vi "Stages and Lasers Control Loop.vi"(8 "error in (no error)":errorcluster, 9 "DataNotifier":refnum<notifier>[](array[refnum]), 10 "DataQueues":refnum<queue>[](array[refnum]), 11 "Message Queues":T1) -> (0 "error out":errorcluster, 1 "DataNotifier Out":refnum<notifier>[](array[refnum]), 2 "DataQueues Out":refnum<queue>[](array[refnum]))   [LabVIEW 2019, in "Acquisition.lvlib"]
doc: "Message loop for handling messages pertaining to the acquisition of data from the hardware."
uses:
  Acquisition.lvlib
  support/Message Queue/All Message Queues.ctl
  support/Message Queue/Message Cluster.ctl
  Settings/Settings.ctl
  HardwareAdapter/Support/Hardware Configuration.ctl
  HardwareAdapter/Support/Camera Configuration.ctl
  <vilib>/userdefined/High Color/IMAQdx.ctl
  Logging/Logging Configuration.ctl
  controls/UI Configuration.ctl
  Acquisition State.ctl
  support/Message Queue/Enqueue Message (Single).vi
  <vilib>/Utility/error.llb/Error Cluster From Error Code.vi
  E:/DevHardSoftware/MMicroscopy/HardwareAdapter/Camera/Dependencies/PVCamNET.dll
  HardwareAdapter/Camera/Dependencies/PVCamNET.dll
  E:/DevHardSoftware/MMicroscopy/HardwareAdapter/Lasers/Dependencies/Oxxius_Boxx.dll
  HardwareAdapter/Lasers/Dependencies/Oxxius_Boxx.dll
  <vilib>/ErrorRing/Error Ring.xnode
  support/Message Queue/Message Queue.lvlib
  Logging/Logging.lvlib
  Settings/Settings.lvlib
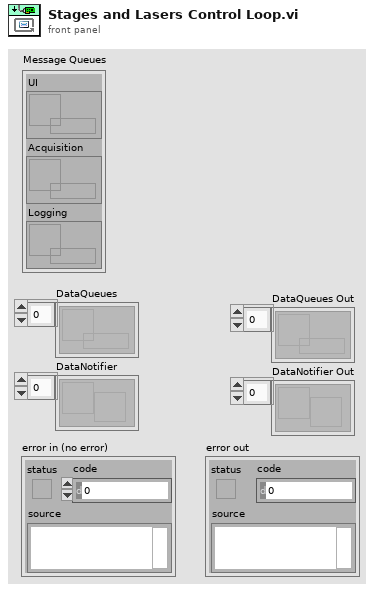
[diagram p1: front panel]
types:
  T1 = typedef "Message Queue.lvlib/All Message Queues.ctl" = cluster{"UI":refnum<queue>, "Acquisition":refnum<queue>, "Logging":refnum<queue>}
  T2 = typedef "Settings.lvlib/Settings.ctl" = cluster{"Hardware Configuration":T3, "Logging Configuration":T6, "HardWare Status":cluster{"CameraAndStages":T7, "Lasers":cluster{"IsConnected":cluster{"405":bool, "488":bool, "532":bool, "561":bool, "647":bool, "785":bool}, "IsOpened":cluster{"405":bool, "488":bool, "532":bool, "561":bool, "647":bool, "785":bool}}}}
  T3 = typedef "Hardware Configuration.ctl" = cluster{"Camera Configuration":T4, "SimpleCamera Configuration":cluster{"Resource":cluster{"Session Out":T5}}, "Stages Configuration":cluster{"Resource":cluster{"NanoStage Ref":i32, "MicroStage Ref":i32, "TirfLock Ref":i32}, "SettingValues":cluster{"NanoState":cluster{"Time":dbl, "X":dbl, "Y":dbl, "Z":dbl}, "MicroState":cluster{"Time 2":dbl, "Z":dbl}, "TirfLock":cluster{"Time":dbl, "X":dbl, "Y":dbl, "Sum":dbl, "Calbrate":dbl}}}, "Lasers Configuration":cluster{"SettingValues":cluster{"405 Power":sgl, "488 Power":sgl, "532 Power":sgl, "561 Power":sgl, "647 Power":sgl, "785 Power":sgl}, "Resource":cluster{"Library Ref":refnum<k24>, "Lasers Ref":cluster{"405 Ref":refnum<k24>, "488 Ref":refnum<k24>, "532 Ref":refnum<k24>, "561 Ref":refnum<k24>, "647 Ref":refnum<k24>, "785 Ref":refnum<k24>}}}}
  T4 = typedef "Camera Configuration.ctl" = cluster{"Resource":cluster{"CameraRef":refnum<k24>, "LibraryRef":refnum<k24>}, "Setting":cluster{"Expouse":dbl}}
  T5 = typedef "IMAQdx.ctl" = refnum<k21>
  T6 = typedef "Logging.lvlib/Logging Configuration.ctl" = cluster{"Log File Base Path":path}
  T7 = typedef "UI Configuration.ctl" = cluster{"Camera":bool, "NanoStage":bool, "MicroStage":bool, "TIRFLock":bool}
  T8 = typedef "Acquisition.lvlib/Acquisition State.ctl" = enum16{"Idle", "Acquiring"}
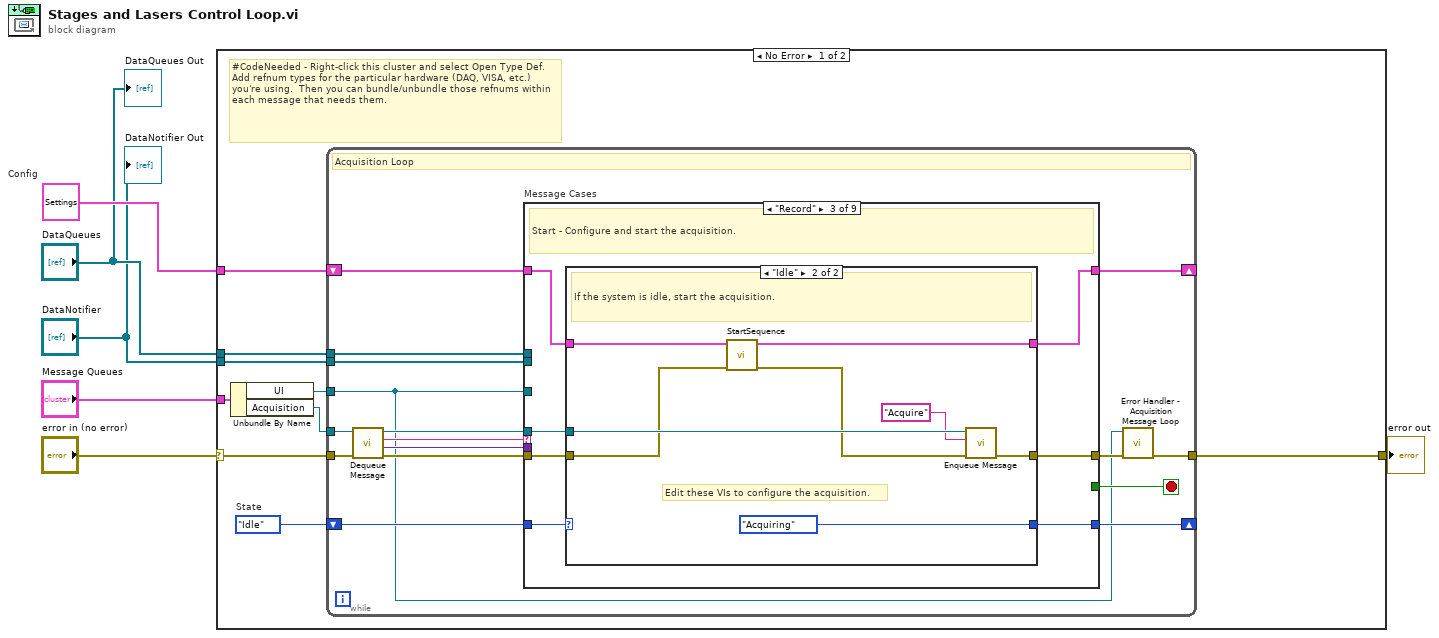
[diagram p0: block diagram]
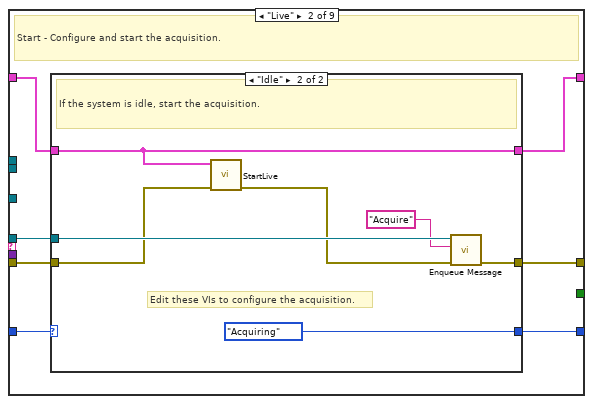
[diagram p3: hidden frame]
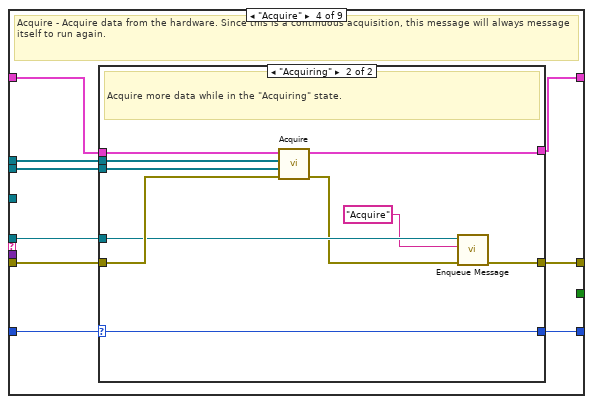
[diagram p6: hidden frame]
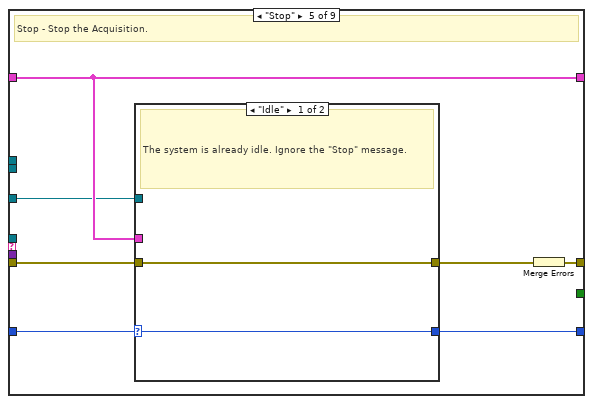
[diagram p8: hidden frame]
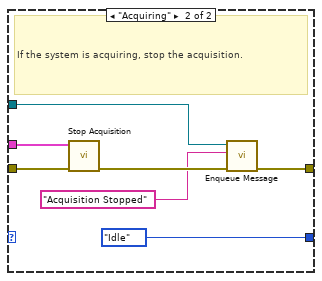
[diagram p9: hidden frame]
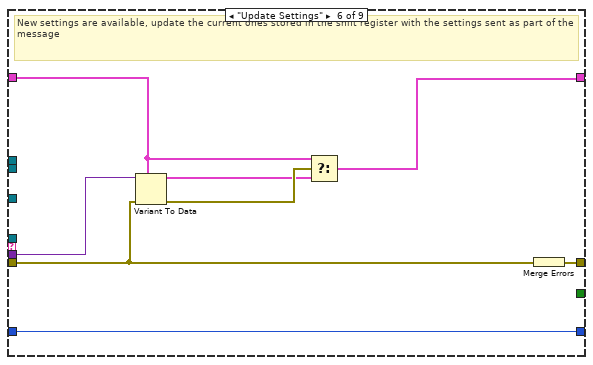
[diagram p10: hidden frame]
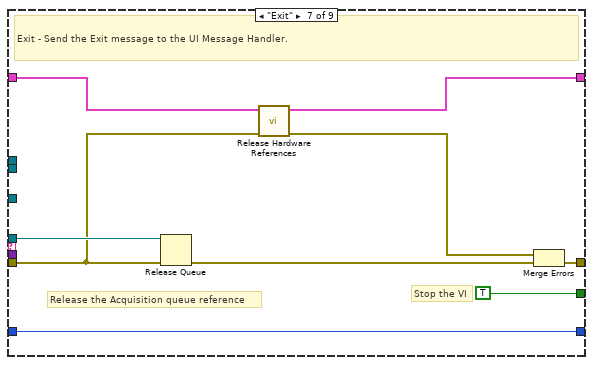
[diagram p11: hidden frame]
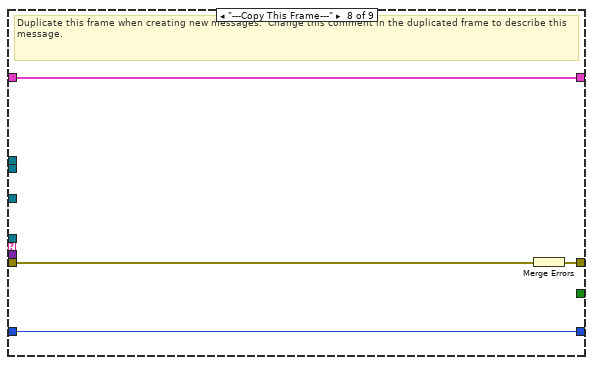
[diagram p12: hidden frame]
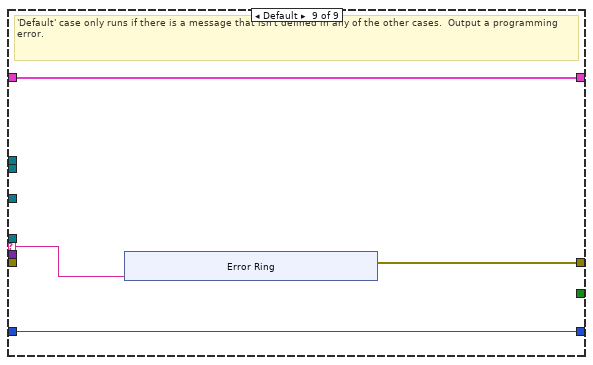
[diagram p13: hidden frame]
diagram:
  w3 = T2 {"Hardware Configuration"={"Camera Configuration"={"Resource"={"CameraRef"=refnum, "LibraryRef"=refnum}, "Setting"={"Expouse"=0.0}}, "SimpleCamera Configuration"={"Resource"={"Session Out"=""}}, "Stages Configuration"={"Resource"={"NanoStage Ref"=0, "MicroStage Ref"=0, "TirfLock Ref"=0}, "SettingValues"={"NanoState"={"Time"=0.0, "X"=0.0, "Y"=0.0, "Z"=0.0}, "MicroState"={"Time 2"=0.0, "Z"=0.0}, "TirfLock"={"Time"=0.0, "X"=0.0, "Y"=0.0, "Sum"=0.0, "Calbrate"=0.0}}}, "Lasers Configuration"={"SettingValues"={"405 Power"=0.0, "488 Power"=0.0, "532 Power"=0.0, "561 Power"=0.0, "647 Power"=0.0, "785 Power"=0.0}, "Resource"={"Library Ref"=refnum, "Lasers Ref"={"405 Ref"=refnum, "488 Ref"=refnum, "532 Ref"=refnum, "561 Ref"=refnum, "647 Ref"=refnum, "785 Ref"=refnum}}}}, "Logging Configuration"={"Log File Base Path"=path ""}, "HardWare Status"={"CameraAndStages"={"Camera"=FALSE, "NanoStage"=FALSE, "MicroStage"=FALSE, "TIRFLock"=FALSE}, "Lasers"={"IsConnected"={"405"=FALSE, "488"=FALSE, "532"=FALSE, "561"=FALSE, "647"=FALSE, "785"=FALSE}, "IsOpened"={"405"=FALSE, "488"=FALSE, "532"=FALSE, "561"=FALSE, "647"=FALSE, "785"=FALSE}}}}  # Config
  n1 = case shown="No Error" "error in (no error)" {
    selector: "error in (no error)" -> [w12 w140]
    tunnel: "Message Queues" -> [w15 _]
    tunnel: [w13 w140] -> w5
    tunnel: "DataQueues" -> [w9 _]
    tunnel: "DataNotifier" -> [w8 _]
    tunnel: w3 -> [w7 _]
    frame No Error {
      w10 = Acquisition_State."Idle"  # State
      # "#CodeNeeded - Right-click this cluster and select Open Type Def.  Add refnum types for the particular hardware (DAQ, VISA, etc.) you're using.  Then you can bundle/unbundle those refnums within each message that needs them."
      n2 = Unbundle By Name(w15) -> ("UI"=w11:refnum<queue>, "Acquisition"=w14:refnum<queue>)
      n3 = while {
        tunnel: w14 -> [w24]
        shift-right: [w30] -> _
        shift-left: w7 -> [w31]
        tunnel: w11 -> [w18]
        shift-right: [w22] -> _
        shift-left: w10 -> [w23]
        tunnel: w12 -> [w28]
        tunnel: [w21] -> w13
        tunnel: w9 -> [w17]
        tunnel: w8 -> [w16]
        stop <- w29 stop-if-true
        # "Acquisition Loop"
        n4 = call "Dequeue Message.vi"("error in (no error)"=w28, "Message Queue"=w24) -> ("error out"=w27:errorcluster, "Message Data"=w25:variant, "Message"=w26:string, "dup Message Queue"=w19:refnum<queue>)  [unwired: 6 in]
        n5 = case "Message Cases" shown="\"Record\"" w26 {
          selector: w26 -> [_ _ _ _ _ _ _ _ w129]
          tunnel: w19 -> [_ w38 w55 w77 _ _ w122 _ _]
          tunnel: w27 -> [w34 w39 w56 w76 w97 w109 w117 w128 _]
          tunnel: [w34 w41 w58 w78 w98 w115 w123 w126 w130] -> w20
          tunnel: w31 -> [w33 w40 w57 w74 w95 w111 w120 w127 w132]
          tunnel: [w33 w37 w54 w75 w95 w110 w116 w127 w132] -> w30
          tunnel: [_ _ _ _ _ _ TRUE _ _] -> w29
          tunnel: w25 -> [_ _ _ _ _ w114 _ _ _]
          tunnel: w18 -> [_ _ _ _ w92 _ _ _ _]
          tunnel: w23 -> [w32 w35 w52 w72 w94 w108 w121 w125 w131]
          tunnel: [w32 w36 w53 w73 w93 w108 w121 w125 w131] -> w22
          tunnel: w17 -> [_ _ _ w71 _ _ _ _ _]
          tunnel: w16 -> [_ _ _ w70 _ _ _ _ _]
          frame "Initialize" {
            # "Initialize  - Initialize is currently a no-op.  The hardware initialization takes place in the 'Start' message."
          }
          frame "Live" {
            # "Start - Configure and start the acquisition."
            n6 = case shown="\"Idle\"" w35 {
              selector: w35 -> [w42 _]
              tunnel: [w43 w45] -> w41
              tunnel: w40 -> [w44 w48]
              tunnel: w39 -> [w43 w47]
              tunnel: w38 -> [_ w51]
              tunnel: [w44 w48] -> w37
              tunnel: [w42 Acquisition_State."Acquiring" ("Acquisition State")] -> w36
              frame "Acquiring" {
                # "The system is already acquiring. Ignore the \"Start\" message."
              }
              frame "Idle" {
                # "Edit these VIs to configure the acquisition."
                # "If the system is idle, start the acquisition."
                n7 = call "StartLive.vi"("error in (no error)"=w47, "Config In"=w48) -> ("error out"=w46:errorcluster)  [unwired: 8 in, 1 out]
                n8 = call-poly "Enqueue Message.vi"("error in (no error)"=w46, "Message"="Acquire", "Message Queue"=w51) -> ("error out"=w45:errorcluster)  [unwired: 7 in, 1 out]
              }
            }
          }
          frame "Record" {
            # "Start - Configure and start the acquisition."
            n9 = case shown="\"Idle\"" w52 {
              selector: w52 -> [w59 _]
              tunnel: [w60 w63] -> w58
              tunnel: w57 -> [w61 w66]
              tunnel: w56 -> [w60 w65]
              tunnel: w55 -> [_ w69]
              tunnel: [w61 w62] -> w54
              tunnel: [w59 Acquisition_State."Acquiring" ("Acquisition State")] -> w53
              frame "Acquiring" {
                # "The system is already acquiring. Ignore the \"Start\" message."
              }
              frame "Idle" {
                # "Edit these VIs to configure the acquisition."
                # "If the system is idle, start the acquisition."
                n10 = call "StartSequence.vi"("error in (no error)"=w65, "Config In"=w66) -> ("error out"=w64:errorcluster, "Config Out"=w62:T2)  [unwired: 8 in]
                n11 = call-poly "Enqueue Message.vi"("error in (no error)"=w64, "Message"="Acquire", "Message Queue"=w69) -> ("error out"=w63:errorcluster)  [unwired: 7 in, 1 out]
              }
            }
          }
          frame "Acquire" {
            # "Acquire - Acquire data from the hardware. Since this is a continuous acquisition, this message will always message itself to run again."
            n12 = case shown="\"Acquiring\"" w72 {
              selector: w72 -> [w79 w90]
              tunnel: [w80 w91] -> w78
              tunnel: w77 -> [_ w84]
              tunnel: w76 -> [w80 w89]
              tunnel: [w81 w85] -> w75
              tunnel: w74 -> [w81 w88]
              tunnel: [w79 w90] -> w73
              tunnel: w71 -> [_ w87]
              tunnel: w70 -> [_ w86]
              frame "Idle" {
                # "Ignore \"Acquire\" messages when the acquisition is idle."
              }
              frame "Acquiring" {
                # "Acquire more data while in the \"Acquiring\" state."
                n13 = call "Acquire.vi"("error in (no error)"=w89, "DataNotifier"=w86, "DataQueues"=w87, "Config In"=w88) -> ("error out"=w83:errorcluster, "Config Out"=w85:T2)  [unwired: 6 in]
                n14 = call-poly "Enqueue Message.vi"("error in (no error)"=w83, "Message"="Acquire", "Message Queue"=w84) -> ("error out"=w91:errorcluster)  [unwired: 7 in, 1 out]
              }
            }
          }
          frame "Stop" {
            # "Stop - Stop the Acquisition."
            n15 = case shown="\"Idle\"" w94 {
              selector: w94 -> [w99 _]
              tunnel: w97 -> [w100 w107]
              tunnel: [w100 w104] -> w96
              tunnel: w95 -> [_ w101]
              tunnel: [w99 Acquisition_State."Idle" ("State")] -> w93
              tunnel: w92 -> [_ w103]
              frame "Idle" {
                # "The system is already idle. Ignore the \"Stop\" message."
              }
              frame "Acquiring" {
                # "If the system is acquiring, stop the acquisition."
                n16 = call "Stop Acquisition.vi"("error in (no error)"=w107, "Config"=w101) -> ("error out"=w106:errorcluster)  [unwired: 9 in]
                n17 = call-poly "Enqueue Message.vi"("error in (no error)"=w106, "Message"="Acquisition Stopped", "Message Queue"=w103) -> ("error out"=w104:errorcluster)  [unwired: 7 in, 1 out]
              }
            }
            n18 = Merge Errors(w96) -> (w98:errorcluster)
          }
          frame "Update Settings" {
            # "New settings are available, update the current ones stored in the shift register with the settings sent as part of the message"
            n19 = Variant To Data(error in=w109, type=w111, Variant=w114) -> (data=w112:T2, error out=w113:errorcluster)
            n20 = Select(t=w111, s=w113, f=w112) -> (s? t:f=w110:T2)
            n21 = Merge Errors(w109) -> (w115:errorcluster)
          }
          frame "Exit" {
            # "Release the Acquisition queue reference"
            # "Stop the VI"
            # "Exit - Send the Exit message to the UI Message Handler."
            n22 = Release Queue(queue=w122, error in (no error)=w117) -> (error out=w119:errorcluster)  [unwired: 1 in, 2 out]
            n23 = call "Release Hardware References.vi"("error in (no error)"=w117, "Config In"=w120) -> ("error out"=w118:errorcluster, "Config Out"=w116:T2)  [unwired: 8 in]
            n24 = Merge Errors(w118, w119) -> (w123:errorcluster)
          }
          frame "---Copy This Frame---" {
            # "Duplicate this frame when creating new messages.  Change this comment in the duplicated frame to describe this message."
            n25 = Merge Errors(w128) -> (w126:errorcluster)
          }
          frame Default {
            # "'Default' case only runs if there is a message that isn't defined in any of the other cases.  Output a programming error."
            n26 = xnode "Error Ring"("parameter 0"=w129) -> ("error out"=w130:errorcluster)
          }
        }
        n27 = call "Error Handler - Acquisition Message Loop.vi"("error in (no error)"=w20, "Message Queue"=w18) -> ("dup error in"=w21:errorcluster)  [unwired: 8 in, 1 out]
      }
    }
    frame Error {
    }
  }
  "error out" <- w5
  "DataQueues Out" <- "DataQueues"
  "DataNotifier Out" <- "DataNotifier"
